vi "Get RemIO UI Ref.vi"(8 "error in (no error)":errorcluster, 11 "11178 in":refnum<class "11178.lvclass">) -> (0 "error out":errorcluster, 2 "VI Refnum":refnum<vi>, 3 "11178 out":refnum<class "11178.lvclass">)   [LabVIEW 2016, in "Modules.lvlib" / "11178.lvclass"]
uses:
  11178.lvclass
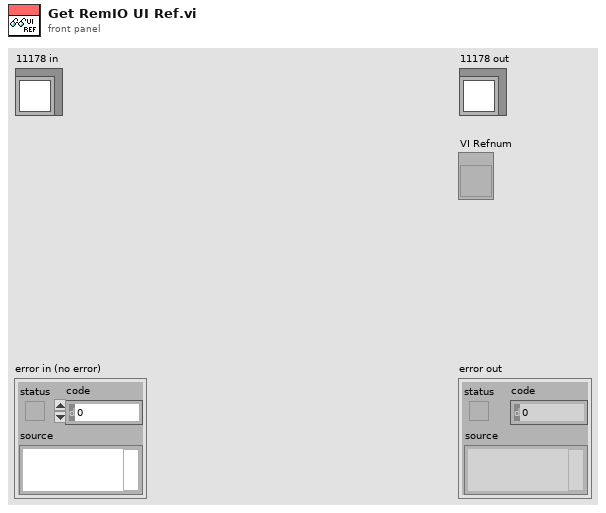
[diagram p1: front panel]
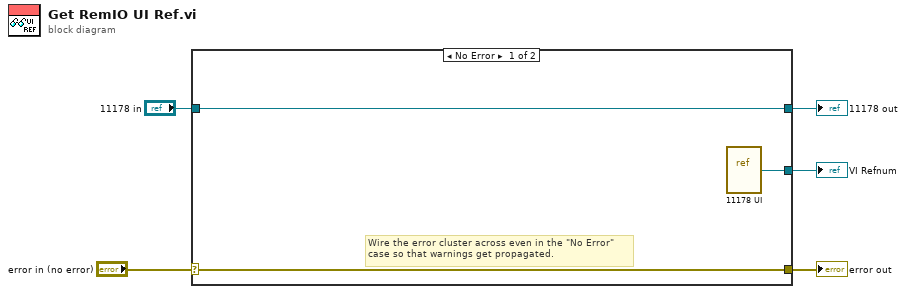
[diagram p0: block diagram]
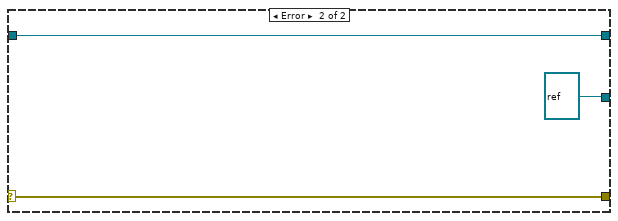
[diagram p2: hidden frame]
diagram:
  n1 = case shown="No Error" "error in (no error)" {
    selector: "error in (no error)" -> [w7 w11]
    tunnel: [w7 w11] -> w1
    tunnel: [w8 w10] -> w3
    tunnel: "11178 in" -> [w8 w10]
    tunnel: [w6 refnum<vi> refnum] -> w2
    frame No Error {
      # "Wire the error cluster across even in the \"No Error\"\ncase so that warnings get propagated."
      n2 = vi-ref "11178 UI.vi"() -> (w6:refnum<vi>)
    }
    frame Error {
    }
  }
  "error out" <- w1
  "11178 out" <- w3
  "VI Refnum" <- w2
